vi "Sub_SetMode.vi"(0 "Mode":u32, 1 "Channel":i32, 2 "Device Handle":u32) -> ()   [LabVIEW 2013]
uses:
  x64_lib/Mightex_LEDDriver_SDK.dll
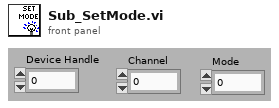
[diagram p1: front panel]
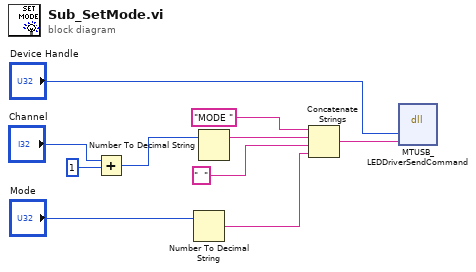
[diagram p0: block diagram]
diagram:
  n1 = Add(x="Channel", y=1) -> (x+y=w1:i32)
  n2 = Number To Decimal String(number="Mode") -> (decimal integer string=w4:string)  [unwired: 1 in]
  n3 = Number To Decimal String(number=w1) -> (decimal integer string=w6:string)  [unwired: 1 in]
  n4 = Concatenate Strings("MODE ", w6, "  ", w4) -> (w9:string)
  n5 = dll-call lib="C:/Users/ignacio/Desktop/Patrick's File Reader Function/led_control/documentation/SDK/x64_lib/Mightex_LEDDriver_SDK.dll" fn="MTUSB_LEDDriverSendCommand"("arg1"="Device Handle", "arg2"=w9) -> ()  [unwired: 6 in, 2 out]
